vi "禹山溶解氧校准.vi"() -> ()   [LabVIEW 2016, in "斯坦道多参数.lvlib"]
uses:
  <vilib>/Utility/miscctls.llb/LVPointTypeDef.ctl
  <vilib>/Analysis/NI_AALBase.lvlib
  <vilib>/Analysis/NI_AALPro.lvlib
  <vilib>/Utility/config.llb/NI_LVConfig.lvlib
panel:
  out "第二点信号值":dbl
  out "第一点信号值":dbl
  out "通讯状态":string
  in  "盐度自动获取":bool
  in  "大气压补偿":dbl format="%#.2f"
  in  "盐度补偿":dbl format="%#.2f"
  out "DO %":dbl caption="饱和度值" format="%#.2f"
  out "第二点校准值":dbl
  out "第一点校准值":dbl
  out "最小值":sgl format="%.2g"
  out "最大值":sgl format="%.2g"
  in  "校准停止":bool
  in  "校准模式":enum16{"两点校准", "单点校准"}(ring)
  in  "标液2":dbl
  in  "标液1":dbl
  out "波形图表":sgl(graph) caption="历史曲线"
  out "温度测量值":dbl caption="温度" format="%#.2f"
  out "变异系数":dbl format="%.6g"
  out "standard deviation":dbl caption="标准差" format="%0.2f"
  out "mean":dbl caption="均值" format="%0.2f"
  out "提示":string
  in  "校准启动":bool
  out "DO mg/L":dbl caption="测试值" format="%#.2f"
  out "电极斜率":dbl format="%#.6f"
  out "电极零点":dbl format="%#.6f"
  # "溶解氧电极设定"
  # "℃"
  # "%"
  # "mg/L"
  # "kPa"
  # "请选择校准模式:"
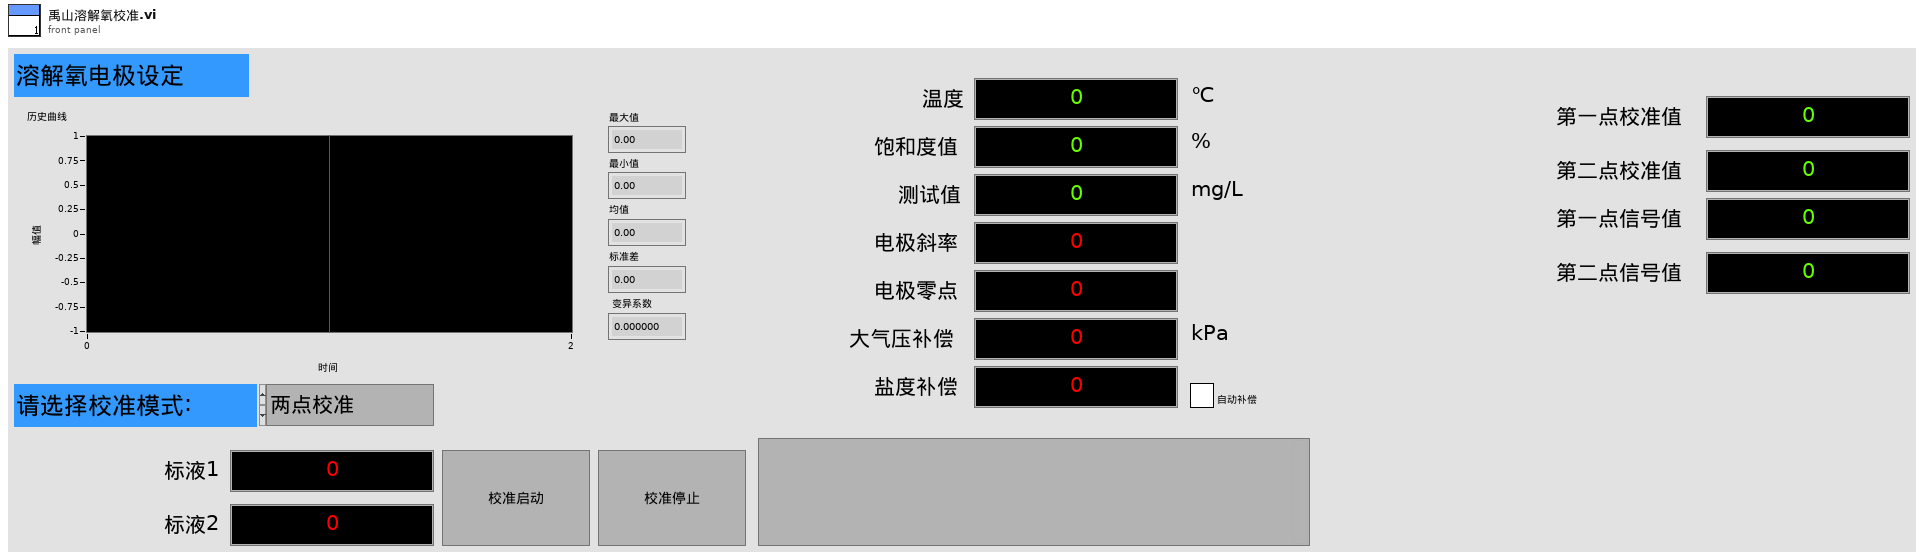
[diagram p1: front panel]
types:
  T1 = typedef "LVPointTypeDef.ctl" = cluster{"Horizontal":i16, "Vertical":i16}
  T2 = typedef "NI_LVConfig.lvlib/Config Data RefNum.ctl" = refnum<k1>
  T3 = enum8{"Enabled", "Disabled", "Disabled and Grayed Out"}
  T4 = cluster{"ph":bool, "DO":bool, "Cond":bool, "Turb":bool, "叶绿素a":bool, "藻密度":bool, "ORP":bool}
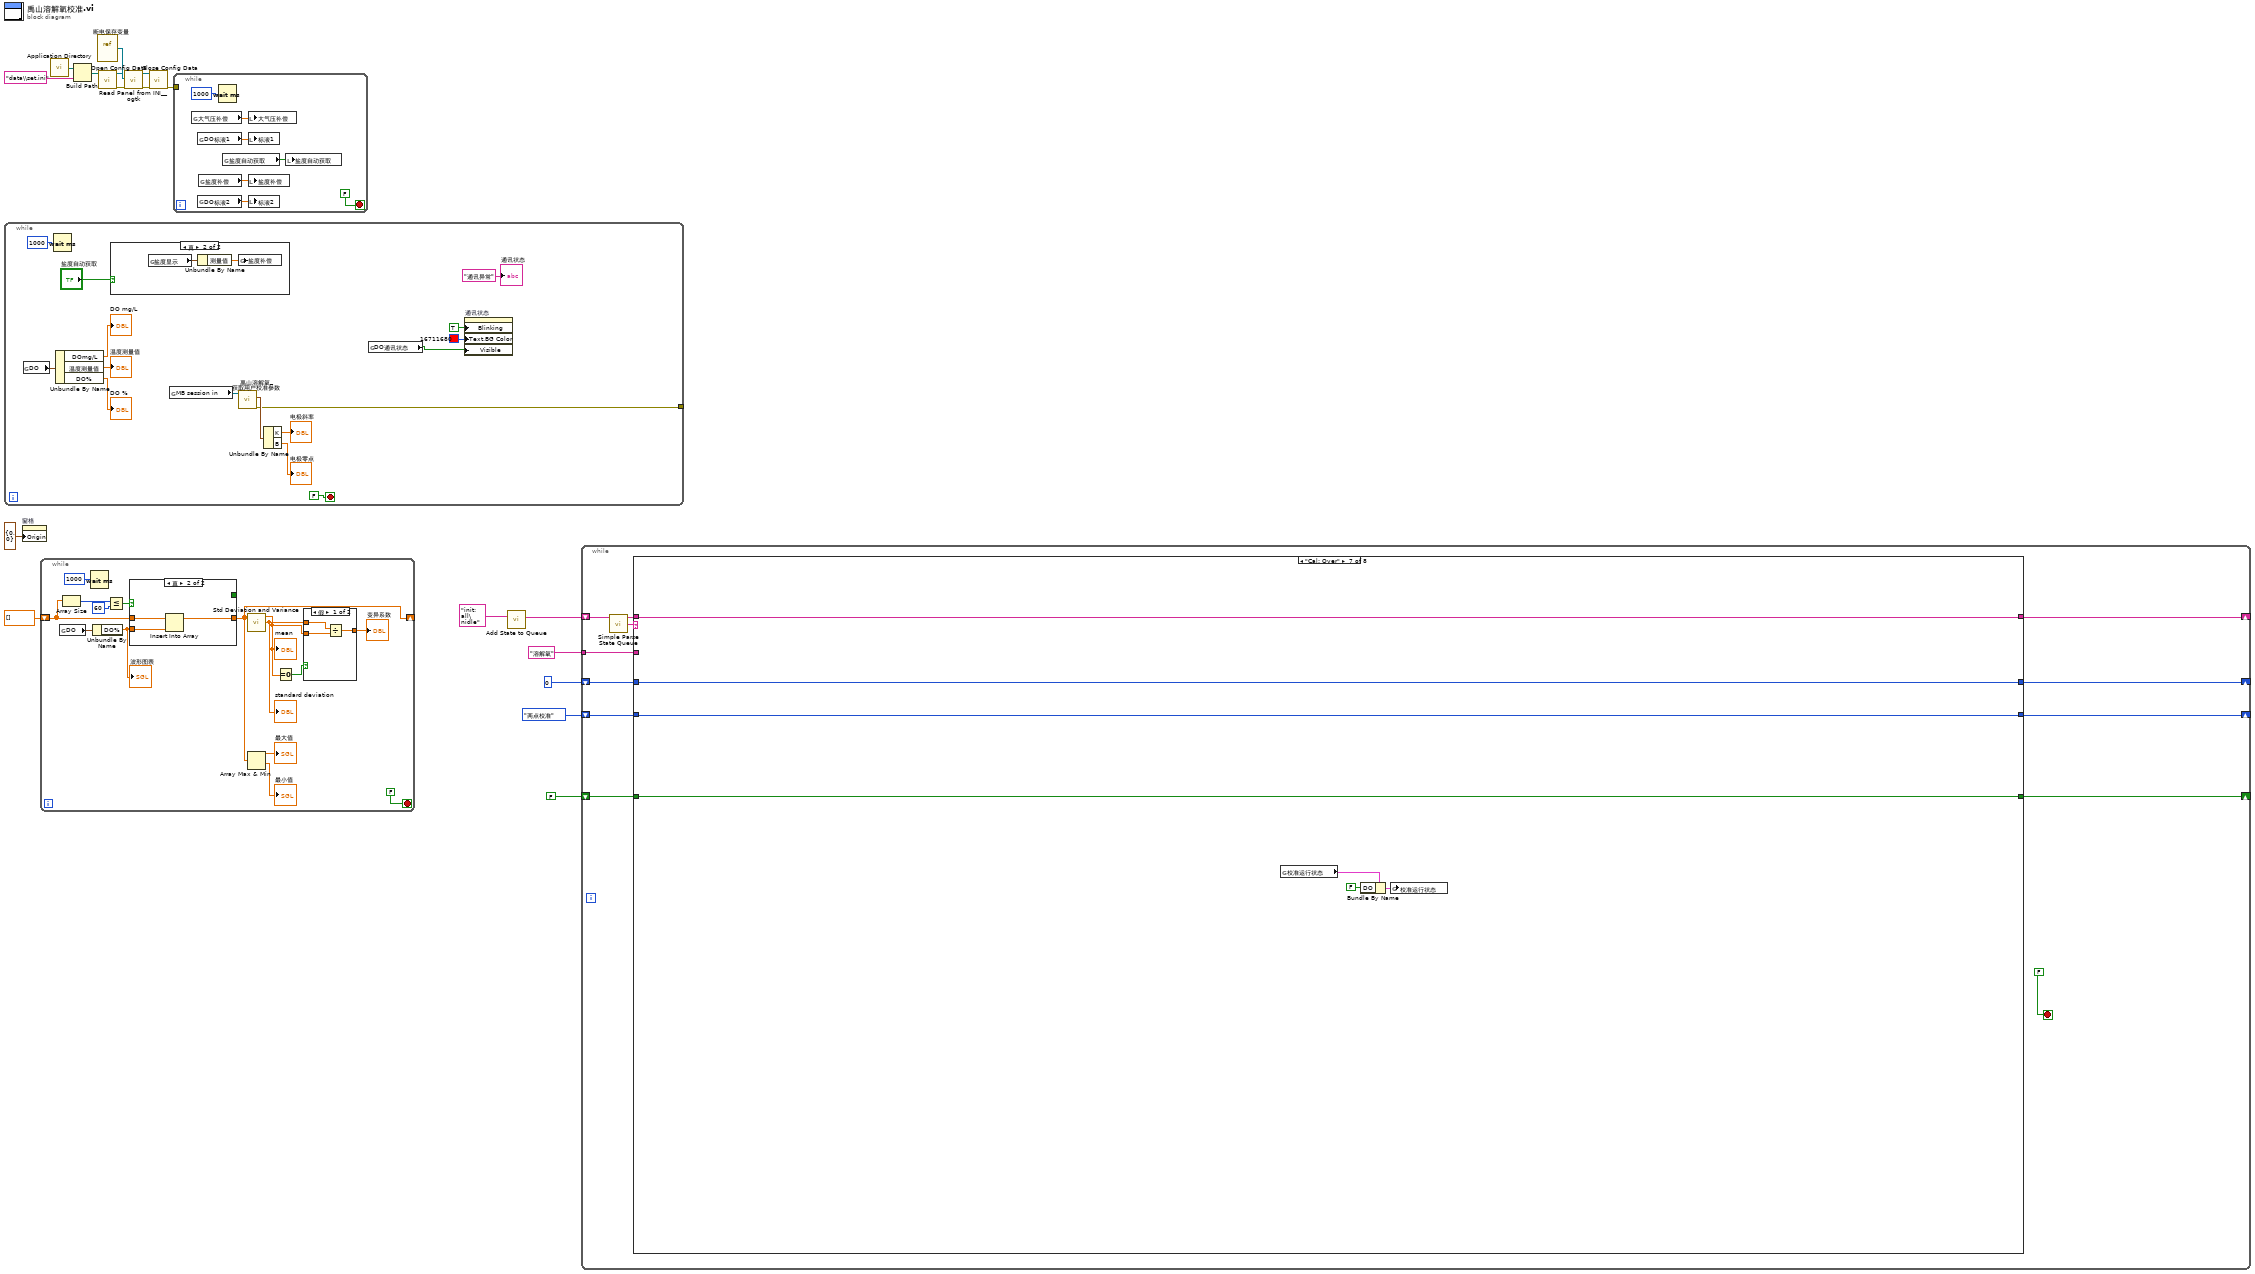
[diagram p0: block diagram]
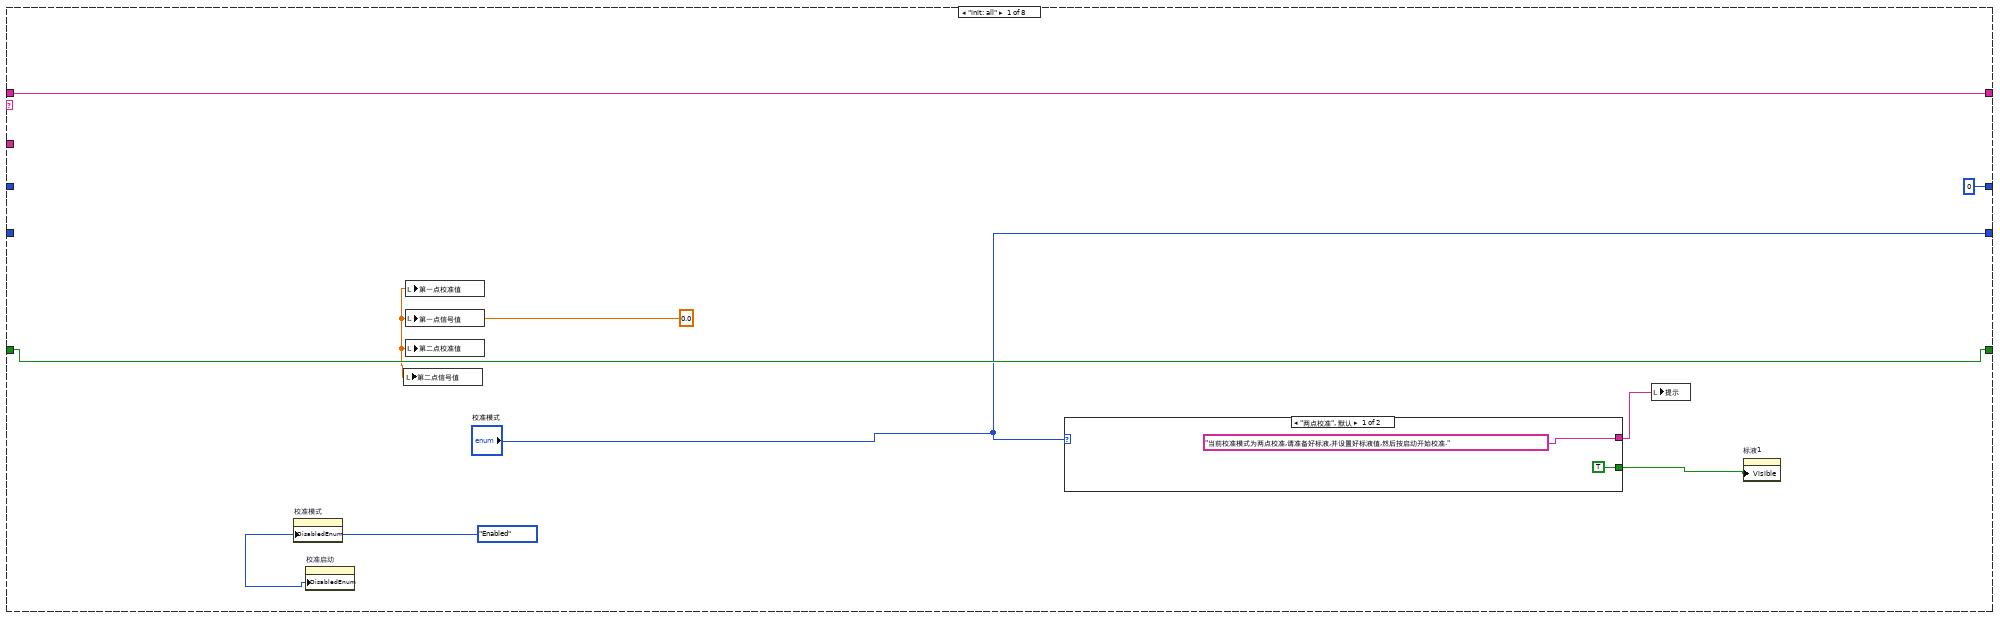
[diagram p2: hidden frame]
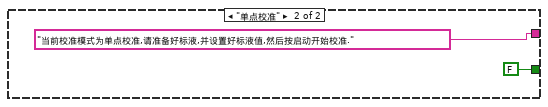
[diagram p3: hidden frame]
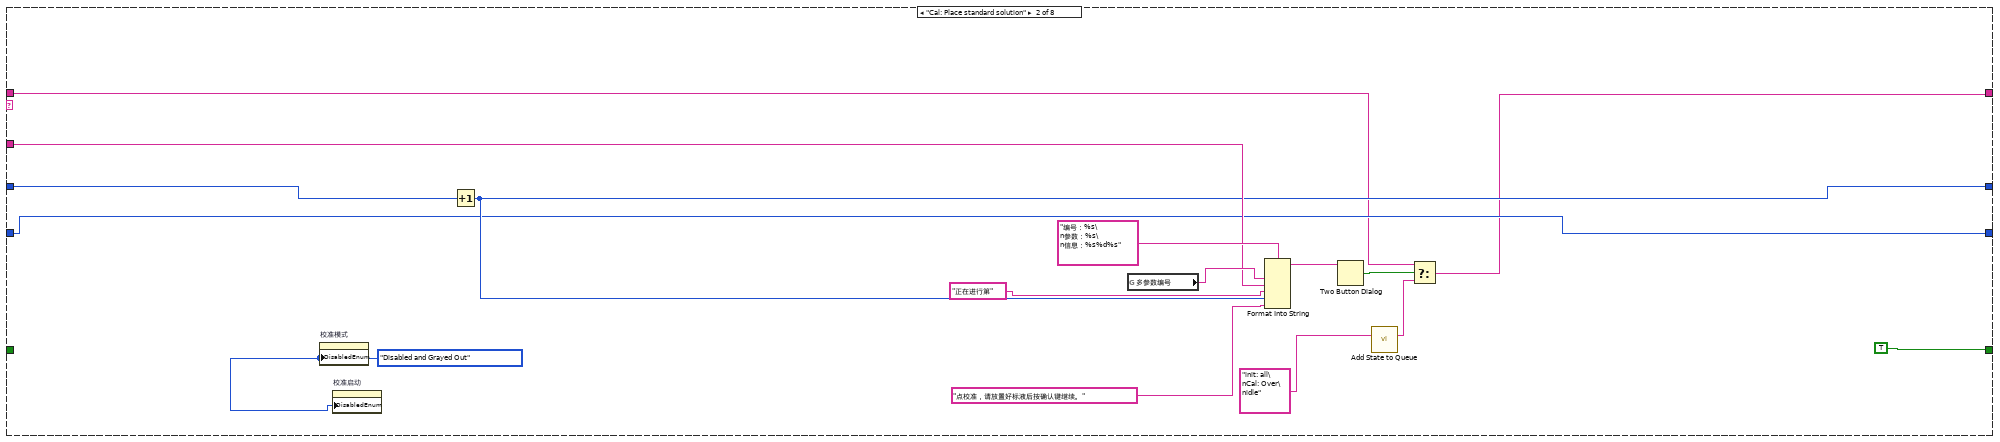
[diagram p4: hidden frame]
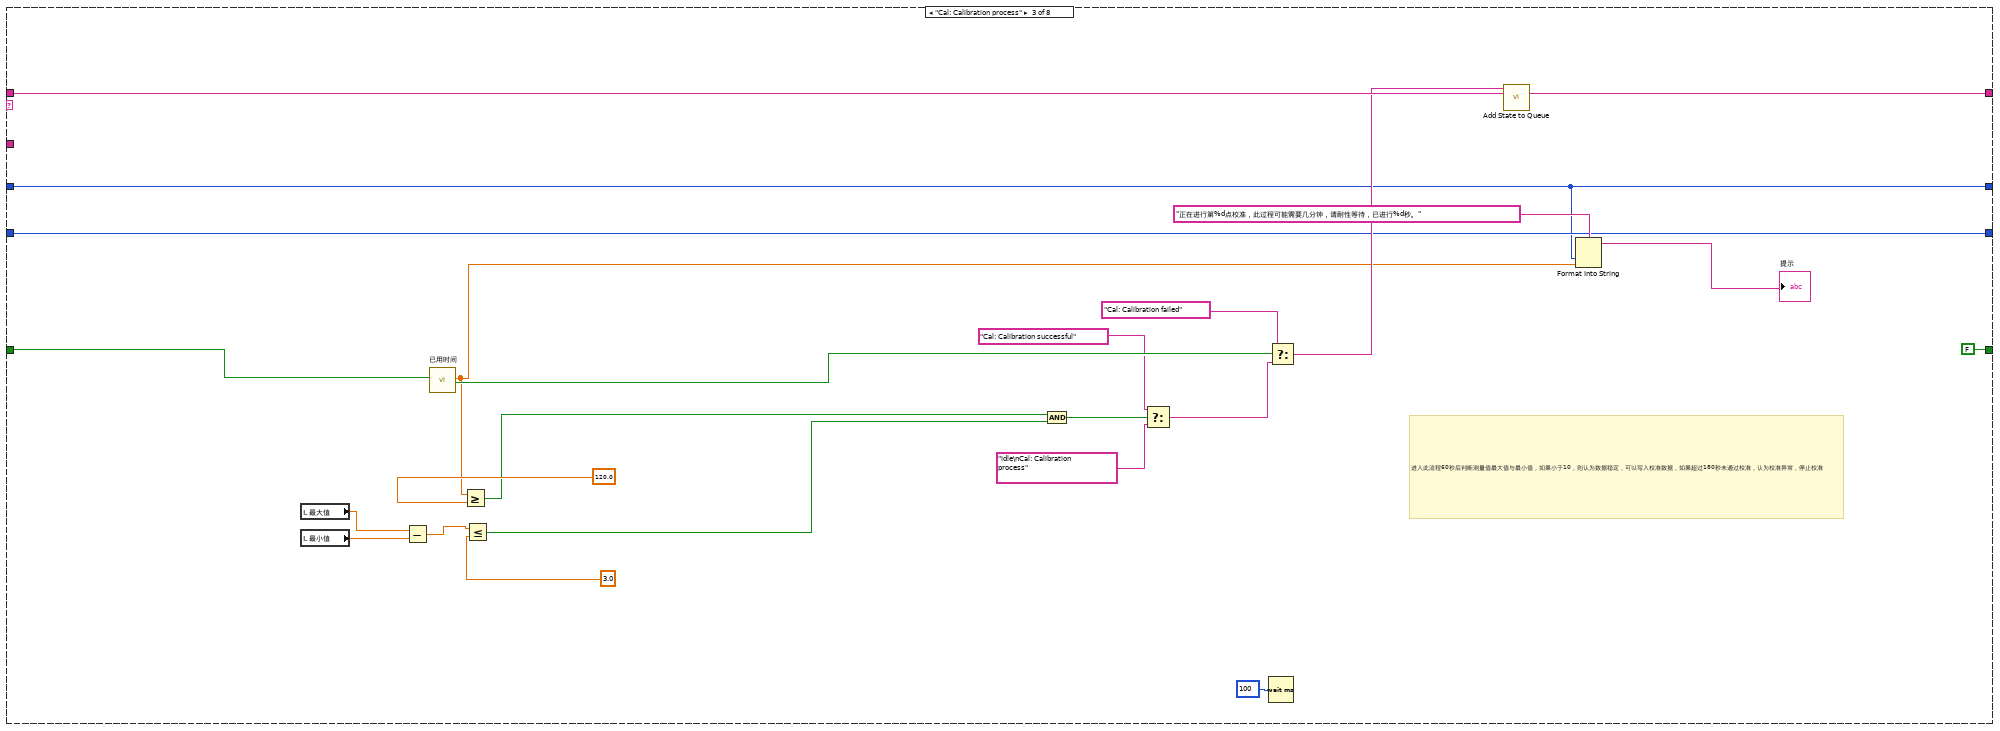
[diagram p5: hidden frame]
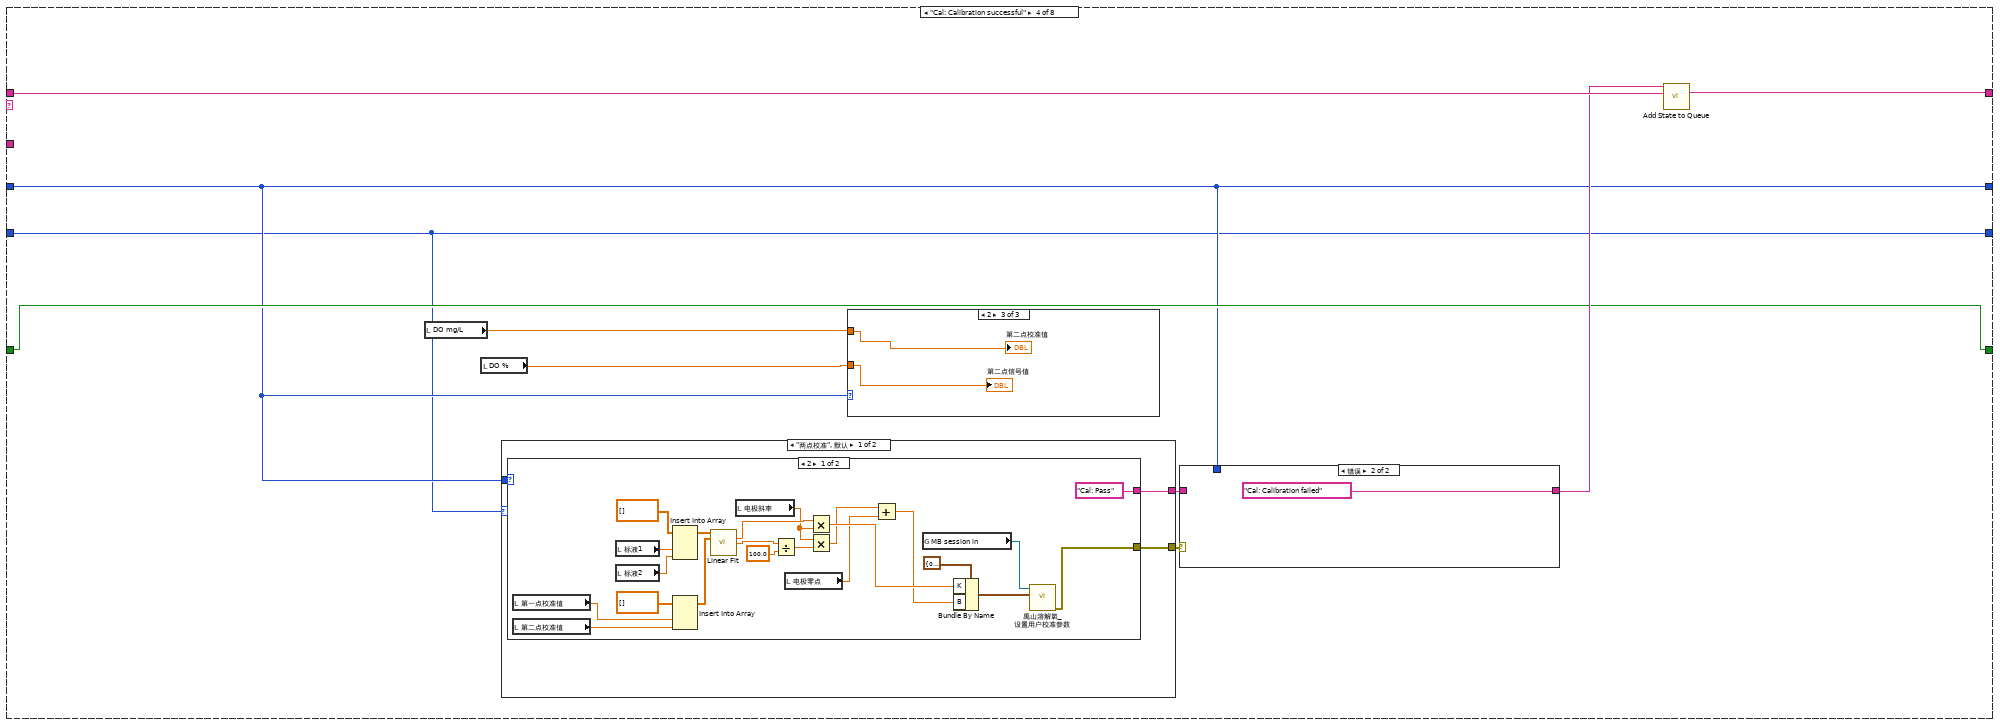
[diagram p6: hidden frame]
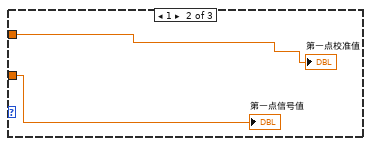
[diagram p8: hidden frame]
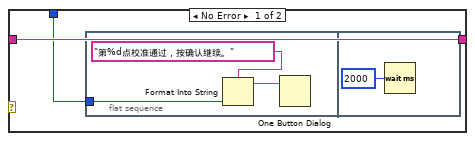
[diagram p9: hidden frame]
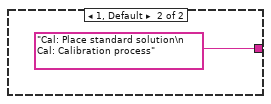
[diagram p10: hidden frame]
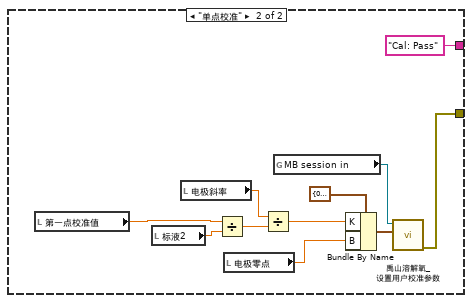
[diagram p11: hidden frame]
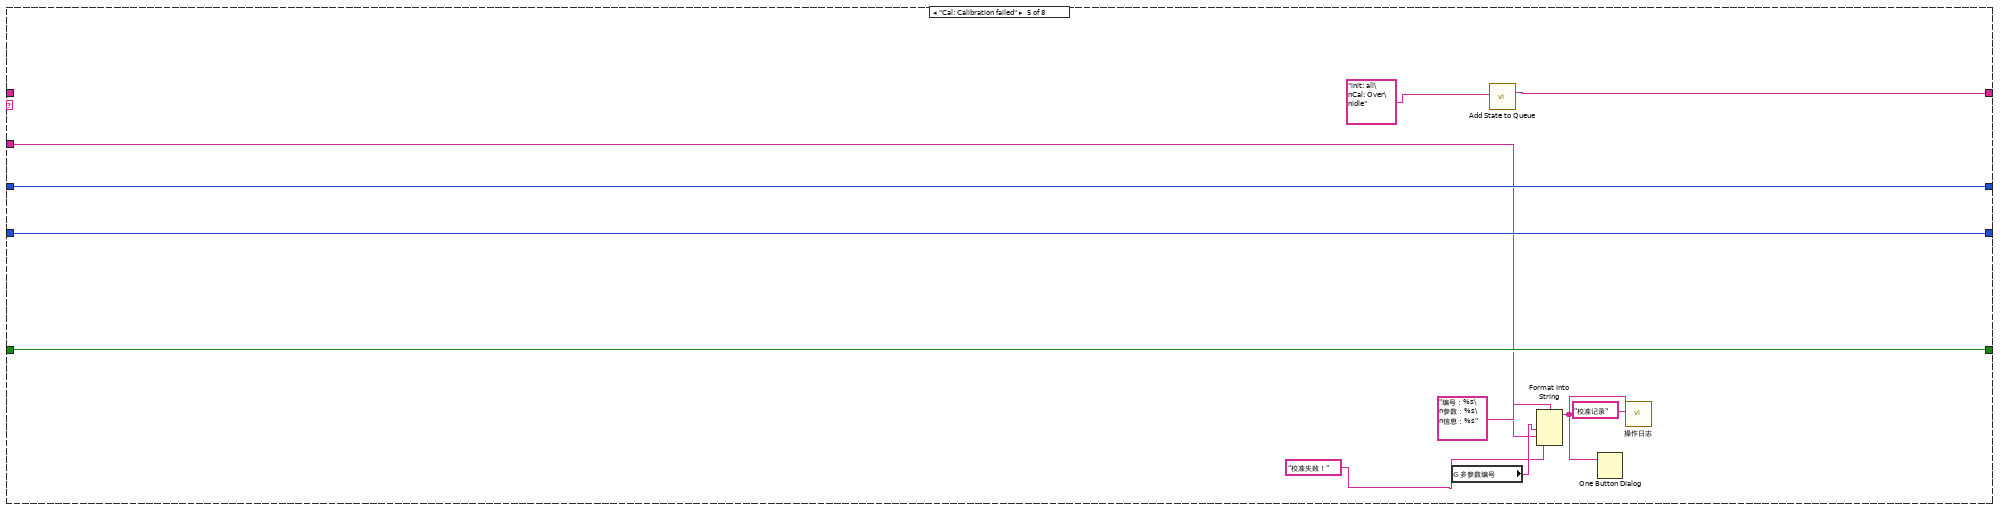
[diagram p12: hidden frame]
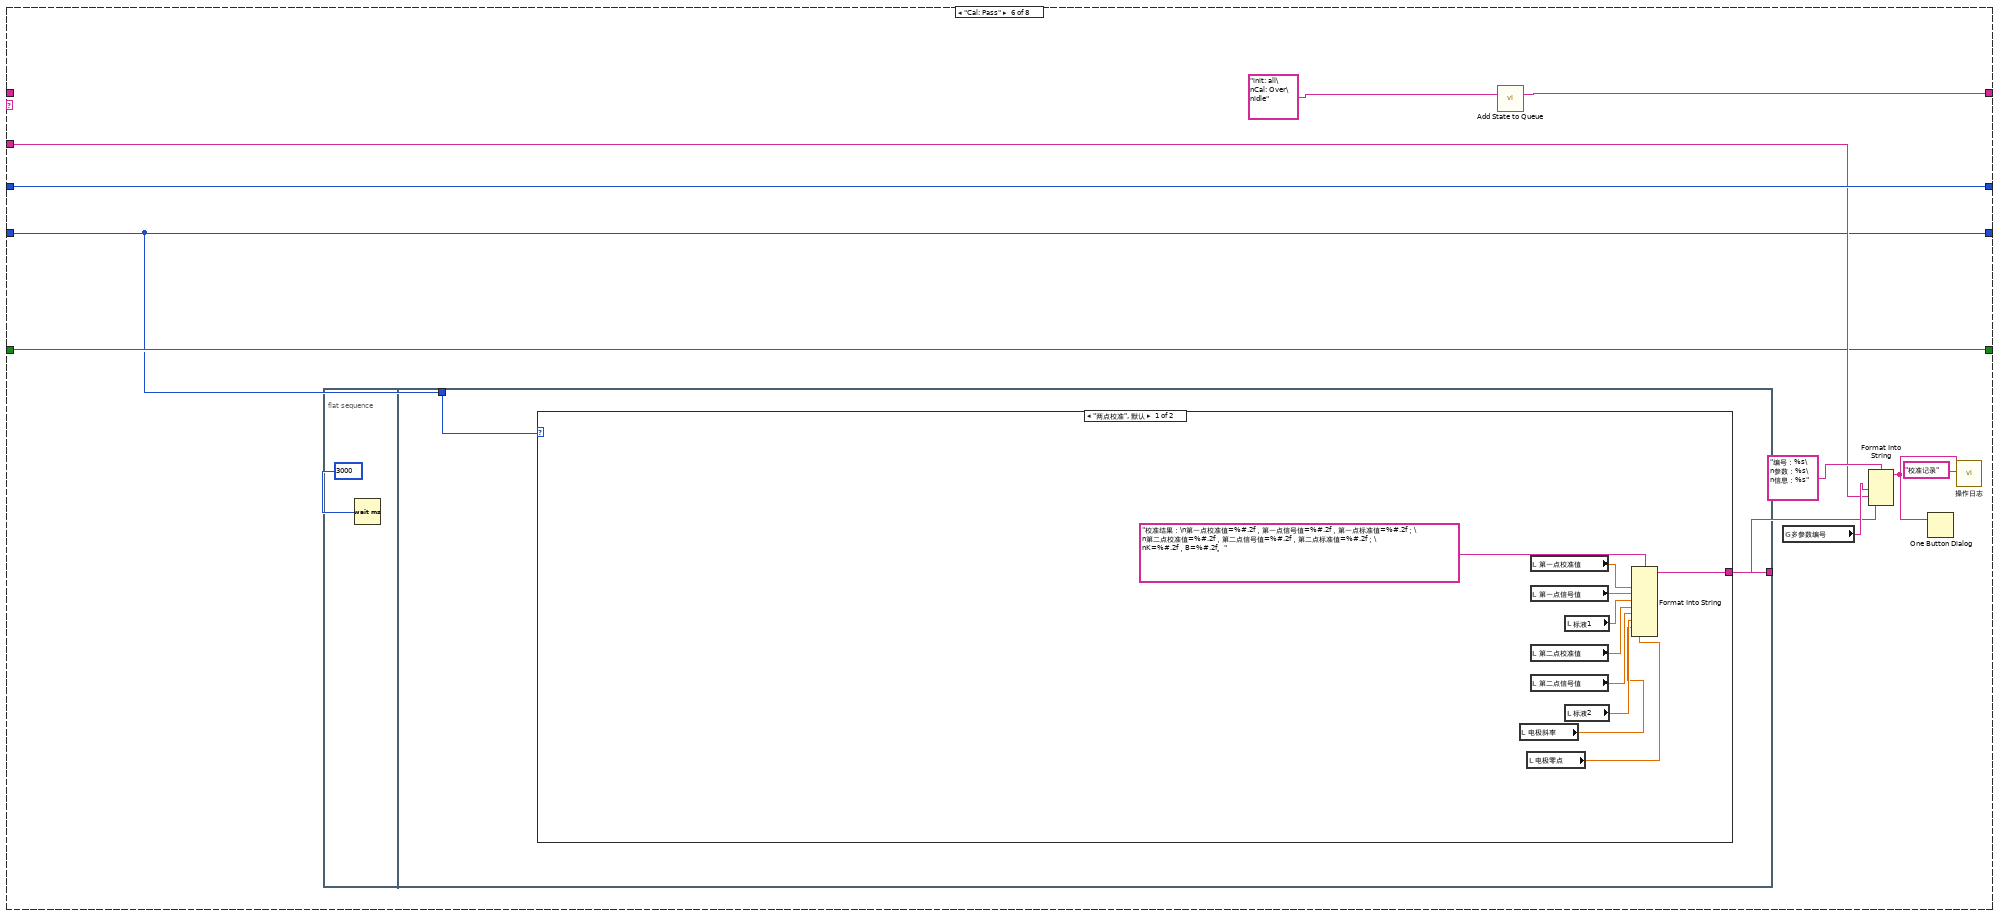
[diagram p13: hidden frame]
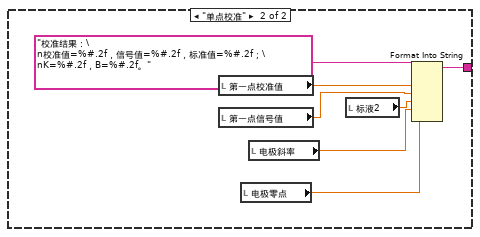
[diagram p14: hidden frame]
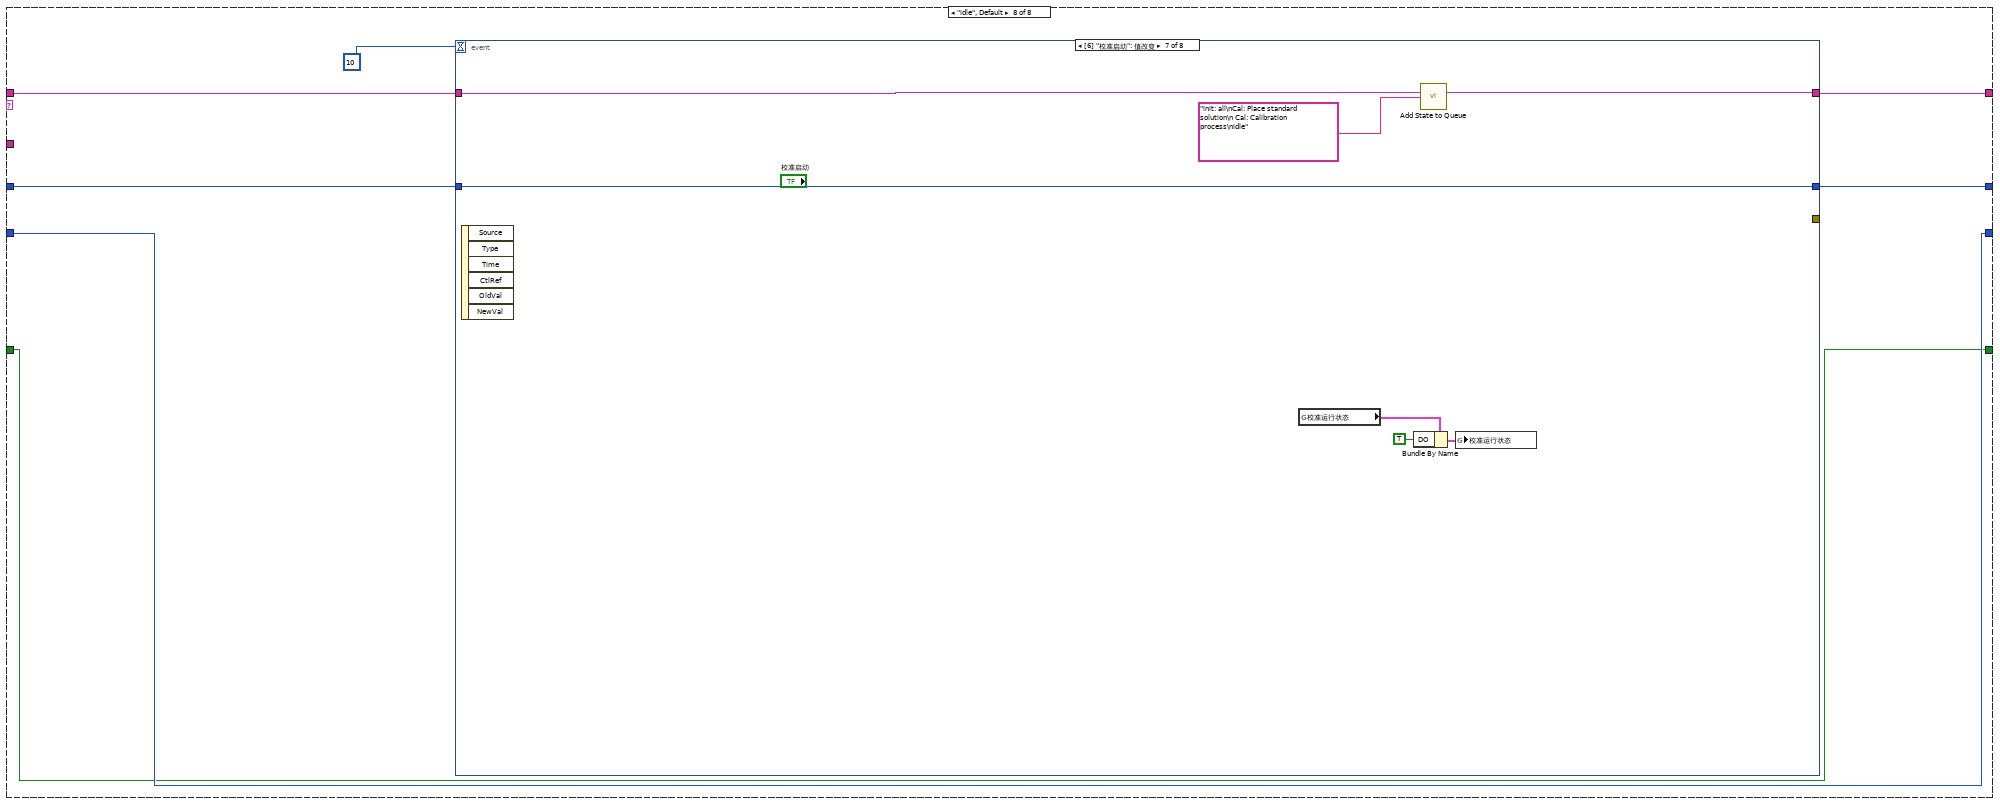
[diagram p15: hidden frame]
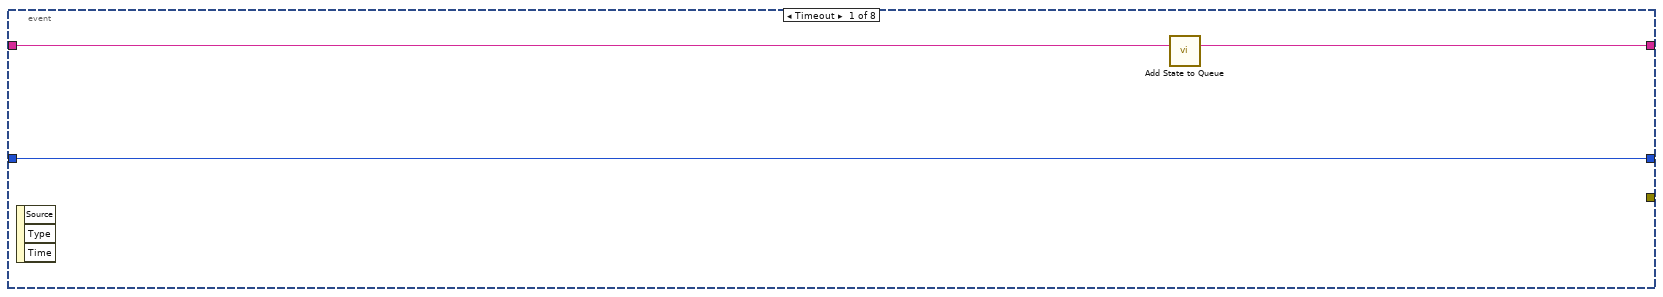
[diagram p16: hidden frame]
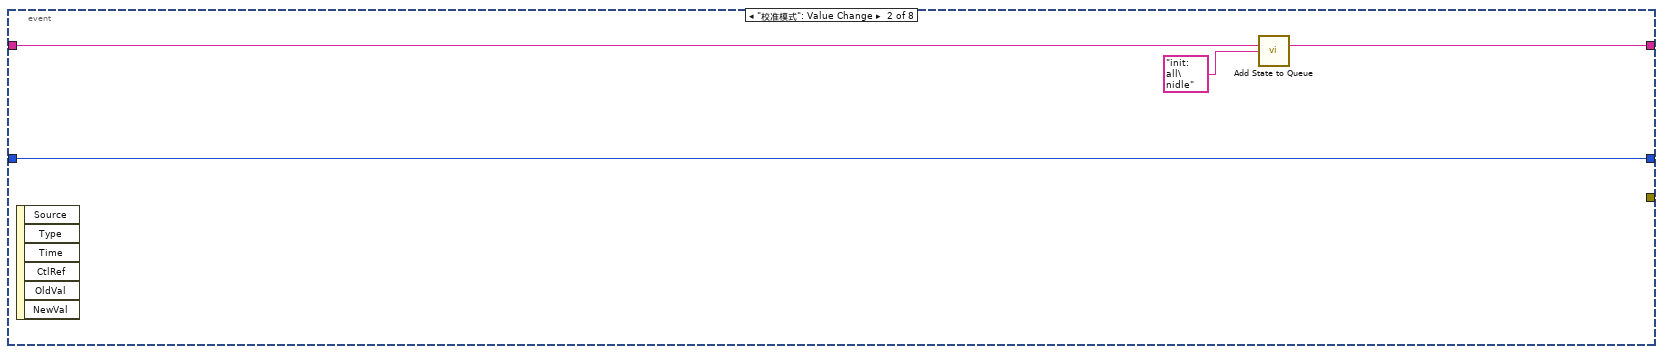
[diagram p17: hidden frame]
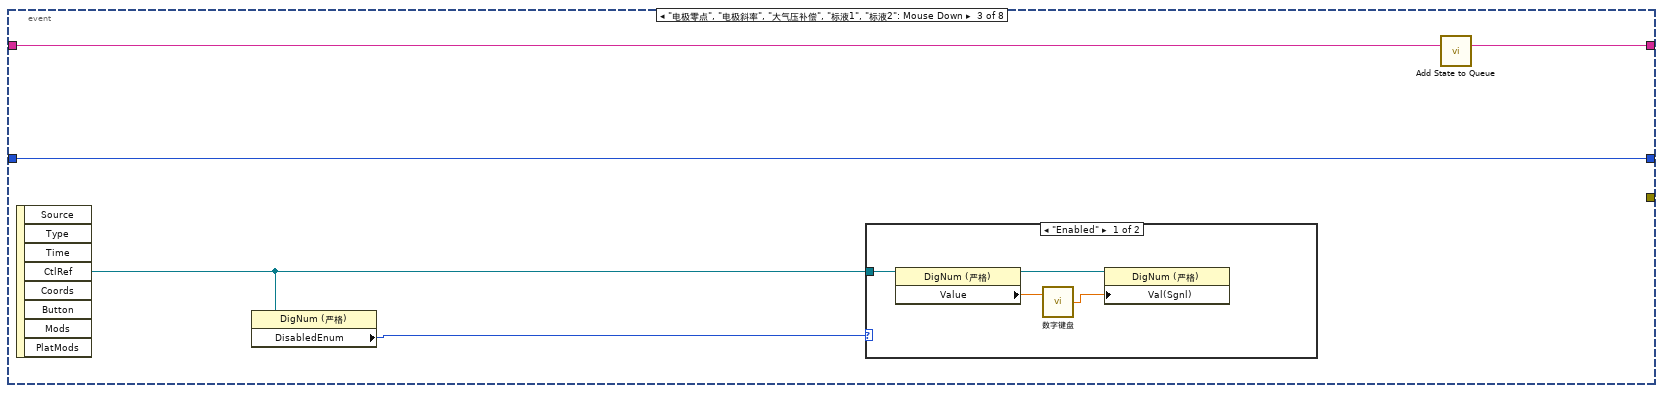
[diagram p18: hidden frame]
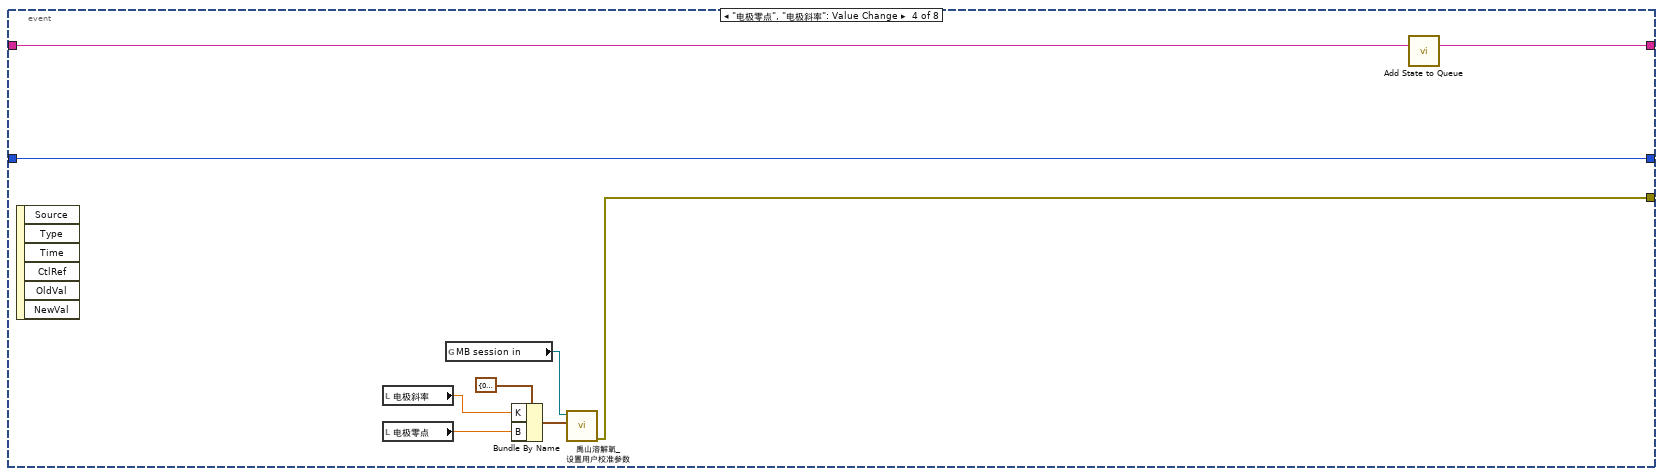
[diagram p20: hidden frame]
diagram:
  n1 = while {
    tunnel: [w28] -> _
    stop <- FALSE stop-if-true
    n2 = global read "禹山过程全局变量.vi" "DO"() -> (w25:cluster{"温度测量值":sgl, "DO%":sgl, "DOmg/L":sgl})
    n3 = Wait (ms)(milliseconds to wait=u32 1000 ("等待时间（毫秒）")) -> ()  [unwired: 1 out]
    n4 = Unbundle By Name(w25) -> ("DOmg/L"=→"DO mg/L":sgl, "温度测量值"=→"温度测量值":sgl, "DO%"=→"DO %":sgl)
    n5 = case shown="真" "盐度自动获取" {
      frame False {
      }
      frame True {
        n6 = global read "多参数全局变量.vi" "盐度显示"() -> (w35:cluster{"温度测量值":sgl, "测量值":sgl, "温度偏移修正值":sgl})
        n7 = Unbundle By Name(w35) -> ("测量值"=w34:sgl)
        n8 = global write "断电保存变量.vi" "盐度补偿"(w34) -> ()
      }
    }
    n9 = global read "多参数全局变量.vi" "MB session in"() -> (w24:refnum<class "MB_Master.lvclass">)
    n10 = call "禹山溶解氧_获取用户校准参数.vi"("MB session in"=w24) -> ("error out"=w28:errorcluster, "输出值"=w31:cluster{"K":sgl, "B":sgl})  [unwired: 8 in, 1 out]
    n11 = Unbundle By Name(w31) -> ("K"=→"电极斜率":sgl, "B"=→"电极零点":sgl)
    n12 = global read "多参数全局变量.vi" "DO通讯状态"() -> (w18:bool)
    n13 = property on="通讯状态" class="Str"("Blinking"=TRUE ("闪烁"), "Text.BG Color"=u32 16711680, "Visible"=w18) -> ()  [unwired: 2 in, 2 out]
    "通讯状态" <- "通讯异常" ("当前串口")
  }
  n14 = property on="窗格" class="Pane"("Origin"=T1 {"Horizontal"=0, "Vertical"=0} ("原点")) -> ()  [unwired: 2 in, 2 out]
  n15 = while {
    shift-right: [w38] -> _
    shift-left: sgl[] [] -> [w46]
    stop <- FALSE stop-if-true
    n16 = global read "禹山过程全局变量.vi" "DO"() -> (w40:cluster{"温度测量值":sgl, "DO%":sgl, "DOmg/L":sgl})
    n17 = Array Size(array=w46) -> (size(s)=w48:i32)
    n18 = Wait (ms)(milliseconds to wait=u32 1000 ("等待时间（毫秒）")) -> ()  [unwired: 1 out]
    n19 = Unbundle By Name(w40) -> ("DO%"=w39:sgl)
    "波形图表" <- w39
    n20 = Less Or Equal?(x=w48, y=60) -> (x <= y?=w47:bool)
    n21 = case shown="真" w47 {
      tunnel: w46 -> [w59 w62]
      tunnel: w39 -> [w57 w61]
      tunnel: [w55 w60] -> w38
      tunnel: [TRUE _] -> _
      frame False {
        n22 = Replace Array Subset(array=w59, new element=w57) -> (w58:sgl[])  [unwired: 1 in]
        n23 = Rotate 1D Array(1:w58, 2:-1 ("n")) -> (0:w55:sgl[])
      }
      frame True {
        n24 = Insert Into Array(array=w62, new element=w61) -> (w60:sgl[])  [unwired: 1 in]
      }
    }
    n25 = call <vilib>:"Std Deviation and Variance.vi"("X"=w38) -> ("mean"=w41:dbl, "standard deviation"=w42:dbl)  [unwired: 1 in, 1 out]
    "standard deviation" <- w42
    "mean" <- w41
    n26 = Array Max & Min(array=w38) -> (max value=→"最大值":sgl, min value=→"最小值":sgl)  [unwired: 2 out]
    n27 = Equal To 0?(x=w41) -> (x = 0?=w45:bool)
    n28 = case shown="假" w45 {
      tunnel: w42 -> [w53 _]
      tunnel: [w52 _] -> w44
      tunnel: w41 -> [w51 _]
      frame False {
        n29 = Divide(x=w53, y=w51) -> (x/y=w52:dbl)
      }
      frame True {
      }
    }
    "变异系数" <- w44
  }
  n30 = call <vilib>:"Application Directory.vi"() -> ("Application Directory"=w12:path)
  n31 = Build Path(base path=w12, name or relative path="data\\set.ini" ("名称或相对路径")) -> (appended path=w13:path)
  n32 = vi-ref "断电保存变量.vi"() -> (w15:refnum<vi>)
  n33 = call <vilib>:"Open Config Data.vi"("configuration file path"=w13) -> ("error out"=w9:errorcluster, "refnum"=w8:T2)  [unwired: 8 in, 1 out]
  n34 = call <userlib>:"Read Panel from INI__ogtk.vi"("error in (no error)"=w9, "VI ref"=w15, "refnum"=w8) -> ("error out"=w11:errorcluster, "refnum out"=w10:T2)  [unwired: 7 in]
  n35 = call <vilib>:"Close Config Data.vi"("error in (no error)"=w11, "refnum"=w10) -> ("error out"=w7:errorcluster)  [unwired: 8 in, 1 out]
  n36 = while {
    tunnel: w7 -> [_]
    stop <- FALSE stop-if-true
    n37 = global read "断电保存变量.vi" "大气压补偿"() -> (w65:dbl)
    n38 = global read "断电保存变量.vi" "DO标液1"() -> (w67:dbl)
    n39 = global read "断电保存变量.vi" "DO标液2"() -> (w66:dbl)
    n40 = global read "断电保存变量.vi" "盐度补偿"() -> (w63:dbl)
    n41 = Wait (ms)(milliseconds to wait=u32 1000 ("等待时间（毫秒）")) -> ()  [unwired: 1 out]
    n42 = global read "断电保存变量.vi" "盐度自动获取"() -> (w64:bool)
    n43 = local write "大气压补偿"(w65) -> ()
    n44 = local write "标液1"(w67) -> ()
    n45 = local write "盐度补偿"(w63) -> ()
    n46 = local write "标液2"(w66) -> ()
    n47 = local write "盐度自动获取"(w64) -> ()
  }
  n48 = call "Add State to Queue.vi"("State(s) In (\"\")"="init: all\nidle" ("State(s) In (\"\")")) -> ("States Out"=w5:string)  [unwired: 14 in]
  n49 = while {
    shift-right: [w77] -> _
    shift-left: w5 -> [w81]
    shift-right: [w74] -> _
    shift-left: 0 -> [w76]
    tunnel: "溶解氧" ("State(s) In (\"\")") -> [w75]
    shift-right: [w72] -> _
    shift-left: enum16{"两点校准", "单点校准"}."两点校准" ("校准模式") -> [w73]
    shift-right: [w70] -> _
    shift-left: FALSE -> [w71]
    stop <- FALSE stop-if-true
    n50 = call "Simple Parse State Queue.vi"("State Queue"=w81) -> ("Remain States"=w78:string, "Next State"=w79:string)  [unwired: 13 in]
    n51 = case shown="\"Cal: Over\"" w79 {
      tunnel: w78 -> [w89 w97 w128 w141 _ _ w240 w247]
      tunnel: [w89 w96 w127 w140 w199 w204 w240 w246] -> w77
      tunnel: w76 -> [_ w105 w112 w135 w202 w213 w239 w244]
      tunnel: w75 -> [_ w106 _ _ w193 w209 _ _]
      tunnel: [0 w103 w112 w135 w202 w213 w239 w245] -> w74
      tunnel: w73 -> [_ w102 w113 w134 w201 w205 w238 w243]
      tunnel: ["校准模式" w102 w113 w134 w201 w205 w238 w243] -> w72
      tunnel: w71 -> [w86 _ w115 w136 w200 w208 w237 w241]
      tunnel: [w86 TRUE FALSE w136 w200 w208 w237 w241] -> w70
      frame "init: all" {
        w84 = T3."Enabled" ("禁用")
        w85 = 0.0 ("第一点校准值")
        n52 = property on="校准模式" class="Enum (严格)"("DisabledEnum"=w84) -> ()  [unwired: 2 in, 2 out]
        n53 = property on="校准启动" class="Bool"("DisabledEnum"=w84) -> ()  [unwired: 2 in, 2 out]
        n54 = local write "第二点信号值"(w85) -> ()
        n55 = local write "第一点校准值"(w85) -> ()
        n56 = local write "第一点信号值"(w85) -> ()
        n57 = local write "第二点校准值"(w85) -> ()
        n58 = case shown="\"两点校准\", 默认" "校准模式" {
          tunnel: ["当前校准模式为两点校准,请准备好标液,并设置好标液值,然后按启动开始校准." ("提示") "当前校准模式为单点校准,请准备好标液,并设置好标液值,然后按启动开始校准." ("提示")] -> w88
          tunnel: [TRUE ("可见") FALSE ("可见")] -> w82
          frame "两点校准", Default {
          }
          frame "单点校准" {
          }
        }
        n59 = local write "提示"(w88) -> ()
        n60 = property on="标液1" class="DigNum (严格)"("Visible"=w82) -> ()  [unwired: 2 in, 2 out]
      }
      frame "Cal: Place standard solution" {
        w95 = T3."Disabled and Grayed Out" ("禁用")
        n61 = property on="校准模式" class="Enum (严格)"("DisabledEnum"=w95) -> ()  [unwired: 2 in, 2 out]
        n62 = property on="校准启动" class="Bool"("DisabledEnum"=w95) -> ()  [unwired: 2 in, 2 out]
        n63 = Increment(x=w105) -> (x+1=w103:i32)
        n64 = global read "多参数全局变量.vi" "多参数编号"() -> (w108:string)
        n65 = Format Into String(format string="编号：%s\n参数：%s\n信息：%s%d%s" ("格式字符串"), w108, w106, "正在进行第" ("消息"), w103, "点校准，请放置好标液后按确认键继续。" ("消息")) -> (resulting string=w100:string)  [unwired: 2 in, 1 out]
        n66 = Two Button Dialog(message=w100) -> (T button?=w99:bool)  [unwired: 2 in]
        n67 = call "Add State to Queue.vi"("State(s) In (\"\")"="init: all\nCal: Over\nidle" ("State(s) In (\"\")")) -> ("States Out"=w98:string)  [unwired: 14 in]
        n68 = Select(t=w97, s=w99, f=w98) -> (s? t:f=w96:string)
      }
      frame "Cal: Calibration process" {
        # "进入此流程60秒后判断测量值最大值与最小值，如果小于10，则认为数据稳定，可以写入校准数据，如果超过180秒未通过校准，认为校准异常，停止校准"
        n69 = local read "最大值"() -> (w132:sgl)
        n70 = local read "最小值"() -> (w131:sgl)
        n71 = Subtract(x=w132, y=w131) -> (x-y=w133:sgl)
        n72 = call "已用时间"("Reset"=w115) -> ("Elapsed Time (s)"=w111:dbl, "Time has Elapsed"=w129:bool)  [unwired: 11 in, 6 out]
        n73 = Greater Or Equal?(x=w111, y=120.0) -> (x >= y?=w124:bool)
        n74 = Less Or Equal?(x=w133, y=3.0) -> (x <= y?=w120:bool)
        n75 = And(x=w124, y=w120) -> (x .and. y?=w121:bool)
        n76 = Select(t="Cal: Calibration successful" ("State(s) In (\"\")"), s=w121, f="idle\nCal: Calibration process" ("State(s) In (\"\")")) -> (s? t:f=w119:string)
        n77 = Wait (ms)(milliseconds to wait=u32 100 ("等待时间（毫秒）")) -> ()  [unwired: 1 out]
        n78 = Select(t="Cal: Calibration failed" ("State(s) In (\"\")"), s=w129, f=w119) -> (s? t:f=w118:string)
        n79 = call "Add State to Queue.vi"("State(s) In Front (\"\")"=w118, "State(s) In (\"\")"=w128) -> ("States Out"=w127:string)  [unwired: 13 in]
        n80 = Format Into String(format string="正在进行第%d点校准，此过程可能需要几分钟，请耐性等待，已进行%d秒。" ("格式字符串"), w112, w111) -> (resulting string=→"提示":string)  [unwired: 2 in, 1 out]
      }
      frame "Cal: Calibration successful" {
        n81 = local read "DO mg/L"() -> (w137:dbl)
        n82 = local read "DO %"() -> (w138:dbl)
        n83 = case shown="\"两点校准\", 默认" w134 {
          tunnel: [w157 w181] -> w143
          tunnel: [w156 "Cal: Pass" ("State(s) In (\"\")")] -> w142
          tunnel: w135 -> [w155 _]
          frame "两点校准", Default {
            n84 = case shown="2" w155 {
              tunnel: [w158 _] -> w157
              tunnel: ["Cal: Pass" ("State(s) In (\"\")") "Cal: Place standard solution\n Cal: Calibration process" ("State(s) In (\"\")")] -> w156
              frame 2 {
                n85 = local read "第一点校准值"() -> (w177:dbl)
                n86 = local read "第二点校准值"() -> (w176:dbl)
                n87 = local read "标液1"() -> (w174:dbl)
                n88 = local read "标液2"() -> (w173:dbl)
                n89 = Insert Into Array(array=dbl[] [] ("Weight"), new element #1=w174, new element #2=w173) -> (w172:dbl[])  [unwired: 1 in]
                n90 = Insert Into Array(array=dbl[] [] ("Weight"), new element #1=w177, new element #2=w176) -> (w171:dbl[])  [unwired: 1 in]
                n91 = call <vilib>:"Linear Fit.vi"("Y"=w172, "X"=w171) -> ("slope"=w167:dbl, "intercept"=w164:dbl)  [unwired: 9 in, 3 out]
                n92 = local read "电极斜率"() -> (w165:dbl)
                n93 = Divide(x=w164, y=100.0) -> (x/y=w160:dbl)
                n94 = local read "电极零点"() -> (w162:dbl)
                n95 = Multiply(x=w167, y=w165) -> (x*y=w166:dbl)
                n96 = Multiply(x=w165, y=w160) -> (x*y=w163:dbl)
                n97 = Add(x=w163, y=w162) -> (x+y=w161:dbl)
                n98 = global read "多参数全局变量.vi" "MB session in"() -> (w170:refnum<class "MB_Master.lvclass">)
                n99 = Bundle By Name(cluster=cluster{"K":sgl, "B":sgl} {"K"=0.0, "B"=0.0} ("用户校准参数"), "K"=w166, "B"=w161) -> (w169:cluster{"K":sgl, "B":sgl})
                n100 = call "禹山溶解氧_设置用户校准参数.vi"("用户校准参数"=w169, "MB session in"=w170) -> ("error out"=w158:errorcluster)  [unwired: 8 in, 1 out]
              }
              frame 1, Default {
              }
            }
          }
          frame "单点校准" {
            n101 = local read "第一点校准值"() -> (w186:dbl)
            n102 = local read "标液2"() -> (w185:dbl)
            n103 = local read "电极斜率"() -> (w183:dbl)
            n104 = Divide(x=w186, y=w185) -> (x/y=w182:dbl)
            n105 = local read "电极零点"() -> (w187:dbl)
            n106 = Divide(x=w183, y=w182) -> (x/y=w184:dbl)
            n107 = global read "多参数全局变量.vi" "MB session in"() -> (w190:refnum<class "MB_Master.lvclass">)
            n108 = Bundle By Name(cluster=cluster{"K":sgl, "B":sgl} {"K"=0.0, "B"=0.0} ("用户校准参数"), "K"=w184, "B"=w187) -> (w189:cluster{"K":sgl, "B":sgl})
            n109 = call "禹山溶解氧_设置用户校准参数.vi"("用户校准参数"=w189, "MB session in"=w190) -> ("error out"=w181:errorcluster)  [unwired: 8 in, 1 out]
          }
        }
        n110 = case shown="2" w135 {
          tunnel: w138 -> [_ w145 w147]
          tunnel: w137 -> [_ w144 w146]
          frame 0, Default {
          }
          frame 1 {
            "第一点信号值" <- w145
            "第一点校准值" <- w144
          }
          frame 2 {
            "第二点信号值" <- w147
            "第二点校准值" <- w146
          }
        }
        n111 = case shown="错误" w143 {
          tunnel: w142 -> [w149 _]
          tunnel: [w149 "Cal: Calibration failed" ("State(s) In (\"\")")] -> w139
          tunnel: w135 -> [w148 _]
          frame No Error {
            n112 = flat-sequence {
              tunnel: w148 -> [w150]
              frame #0 {
                n113 = Format Into String(format string="第%d点校准通过，按确认继续。" ("格式字符串"), w150) -> (resulting string=w152:string)  [unwired: 2 in, 1 out]
                n114 = One Button Dialog(message=w152) -> ()  [unwired: 1 in, 1 out]
              }
              frame #1 {
                n115 = Wait (ms)(milliseconds to wait=u32 2000 ("等待时间（毫秒）")) -> ()  [unwired: 1 out]
              }
            }
          }
          frame Error {
          }
        }
        n116 = call "Add State to Queue.vi"("State(s) In Front (\"\")"=w139, "State(s) In (\"\")"=w141) -> ("States Out"=w140:string)  [unwired: 13 in]
      }
      frame "Cal: Calibration failed" {
        n117 = global read "多参数全局变量.vi" "多参数编号"() -> (w196:string)
        n118 = call "Add State to Queue.vi"("State(s) In (\"\")"="init: all\nCal: Over\nidle" ("State(s) In (\"\")")) -> ("States Out"=w199:string)  [unwired: 14 in]
        n119 = Format Into String(format string="编号：%s\n参数：%s\n信息：%s" ("格式字符串"), w196, w193, "校准失败！" ("消息")) -> (resulting string=w195:string)  [unwired: 2 in, 1 out]
        n120 = One Button Dialog(message=w195) -> ()  [unwired: 1 in, 1 out]
        n121 = call "操作日志.vi"("table"="校准记录", "日志信息"=w195) -> ()  [unwired: 9 in, 1 out]
      }
      frame "Cal: Pass" {
        n122 = flat-sequence {
          tunnel: [w216] -> w206
          tunnel: w205 -> [w215]
          frame #0 {
            n123 = Wait (ms)(milliseconds to wait=u32 3000 ("等待时间（毫秒）")) -> ()  [unwired: 1 out]
          }
          frame #1 {
            n124 = case shown="\"两点校准\", 默认" w215 {
              tunnel: [w226 w233] -> w216
              frame "两点校准", Default {
                n125 = local read "电极斜率"() -> (w218:dbl)
                n126 = local read "电极零点"() -> (w217:dbl)
                n127 = local read "第一点校准值"() -> (w224:dbl)
                n128 = local read "第一点信号值"() -> (w225:dbl)
                n129 = local read "第二点校准值"() -> (w221:dbl)
                n130 = local read "第二点信号值"() -> (w220:dbl)
                n131 = local read "标液1"() -> (w222:dbl)
                n132 = local read "标液2"() -> (w219:dbl)
                n133 = Format Into String(format string="校准结果：\n第一点校准值=%#.2f，第一点信号值=%#.2f，第一点标准值=%#.2f；\n第二点校准值=%#.2f，第二点信号值=%#.2f，第二点标准值=%#.2f；\nK=%#.2f，B=%#.2f。" ("提示"), w224, w225, w222, w221, w220, w219, w218, w217) -> (resulting string=w226:string)  [unwired: 2 in, 1 out]
              }
              frame "单点校准" {
                n134 = local read "第一点校准值"() -> (w232:dbl)
                n135 = local read "第一点信号值"() -> (w230:dbl)
                n136 = local read "电极零点"() -> (w227:dbl)
                n137 = local read "电极斜率"() -> (w228:dbl)
                n138 = local read "标液2"() -> (w229:dbl)
                n139 = Format Into String(format string="校准结果：\n校准值=%#.2f，信号值=%#.2f，标准值=%#.2f；\nK=%#.2f，B=%#.2f。" ("提示"), w232, w230, w229, w228, w227) -> (resulting string=w233:string)  [unwired: 2 in, 1 out]
              }
            }
          }
        }
        n140 = call "Add State to Queue.vi"("State(s) In (\"\")"="init: all\nCal: Over\nidle" ("State(s) In (\"\")")) -> ("States Out"=w204:string)  [unwired: 14 in]
        n141 = global read "多参数全局变量.vi" "多参数编号"() -> (w210:string)
        n142 = Format Into String(format string="编号：%s\n参数：%s\n信息：%s" ("格式字符串"), w210, w209, w206) -> (resulting string=w207:string)  [unwired: 2 in, 1 out]
        n143 = One Button Dialog(message=w207) -> ()  [unwired: 1 in, 1 out]
        n144 = call "操作日志.vi"("table"="校准记录", "日志信息"=w207) -> ()  [unwired: 9 in, 1 out]
      }
      frame "Cal: Over" {
        n145 = global read "多参数全局变量.vi" "校准运行状态"() -> (w235:T4)
        n146 = Bundle By Name(cluster=w235, "DO"=FALSE) -> (w236:T4)
        n147 = global write "多参数全局变量.vi" "校准运行状态"(w236) -> ()
      }
      frame "idle", Default {
        n148 = event shown="[6] \"校准启动\": 值改变" {
          selector: _ -> [_ _ _ _ _ _ _ _]
          dyn-events: _ -> [_ _ _ _ _ _ _ _]
          timeout: 10 -> [_ _ _ _ _ _ _ _]
          tunnel: [_ _ _ w265 _ _ _ _] -> _
          tunnel: w247 -> [w250 w254 w257 w264 w273 w295 w310 _]
          tunnel: [w249 w253 w258 w271 w274 w297 w309 w312] -> w246
          tunnel: [w248 w251 w259 w272 w275 w296 w307 w313] -> w245
          tunnel: w244 -> [w248 w251 w259 w272 w275 w296 w307 w313]
          event Timeout {
            n149 = event-data() -> ()  [unwired: 1 in, 3 out]
            n150 = call "Add State to Queue.vi"("State(s) In (\"\")"=w250) -> ("States Out"=w249:string)  [unwired: 14 in]
          }
          event "校准模式": Value Change {
            n151 = event-data() -> ()  [unwired: 1 in, 6 out]
            n152 = call "Add State to Queue.vi"("State(s) In (\"\")"=w254, "State(s) At Back (\"\")"="init: all\nidle" ("State(s) In (\"\")")) -> ("States Out"=w253:string)  [unwired: 13 in]
          }
          event "电极零点", "电极斜率", "大气压补偿", "标液1", "标液2": Mouse Down {
            n153 = event-data() -> ("CtlRef"=w256:refnum<vi>)  [unwired: 1 in, 7 out]
            n154 = property class="DigNum (严格)"(reference=w256) -> ("DisabledEnum"=w255:T3)  [unwired: 1 in, 2 out]
            n155 = case shown="\"Enabled\"" w255 {
              tunnel: w256 -> [w263 _]
              frame "Enabled" {
                n156 = property class="DigNum (严格)"(reference=w263) -> (reference out=w260:refnum<vi>, "Value"=w261:dbl)  [unwired: 1 in, 1 out]
                n157 = call "数字键盘.vi"("OldNumber"=w261) -> ("NewNumber"=w262:dbl)  [unwired: 1 in]
                n158 = property class="DigNum (严格)"(reference=w260, "Val(Sgnl)"=w262) -> ()  [unwired: 1 in, 2 out]
              }
              frame "Disabled", Default {
              }
            }
            n159 = call "Add State to Queue.vi"("State(s) In (\"\")"=w257) -> ("States Out"=w258:string)  [unwired: 14 in]
          }
          event "电极零点", "电极斜率": Value Change {
            n160 = event-data() -> ()  [unwired: 1 in, 6 out]
            n161 = local read "电极斜率"() -> (w268:dbl)
            n162 = local read "电极零点"() -> (w267:dbl)
            n163 = global read "多参数全局变量.vi" "MB session in"() -> (w266:refnum<class "MB_Master.lvclass">)
            n164 = Bundle By Name(cluster=cluster{"K":sgl, "B":sgl} {"K"=0.0, "B"=0.0} ("用户校准参数"), "K"=w268, "B"=w267) -> (w269:cluster{"K":sgl, "B":sgl})
            n165 = call "禹山溶解氧_设置用户校准参数.vi"("用户校准参数"=w269, "MB session in"=w266) -> ("error out"=w265:errorcluster)  [unwired: 8 in, 1 out]
            n166 = call "Add State to Queue.vi"("State(s) In (\"\")"=w264) -> ("States Out"=w271:string)  [unwired: 14 in]
          }
          event "标液1", "标液2", "大气压补偿", "盐度补偿", "盐度自动获取": Value Change {
            n167 = event-data() -> ()  [unwired: 1 in, 6 out]
            n168 = flat-sequence {
              frame #0 {
                n169 = local read "盐度自动获取"() -> (w276:bool)
                n170 = global write "断电保存变量.vi" "盐度补偿"("盐度补偿") -> ()
                n171 = global write "断电保存变量.vi" "DO标液1"("标液1") -> ()
                n172 = global write "断电保存变量.vi" "DO标液2"("标液2") -> ()
                n173 = global write "断电保存变量.vi" "大气压补偿"("大气压补偿") -> ()
                n174 = global write "断电保存变量.vi" "盐度自动获取"(w276) -> ()
              }
              frame #1 {
                n175 = call <vilib>:"Application Directory.vi"() -> ("Application Directory"=w290:path)
                n176 = Build Path(base path=w290, name or relative path="data\\set.ini" ("名称或相对路径")) -> (appended path=w289:path)
                n177 = call <vilib>:"Open Config Data.vi"("configuration file path"=w289) -> ("error out"=w293:errorcluster, "refnum"=w294:T2)  [unwired: 8 in, 1 out]
                n178 = vi-ref "断电保存变量.vi"() -> (w287:refnum<vi>)
                n179 = call <userlib>:"Write Panel to INI__ogtk.vi"("error in (no error)"=w293, "VI ref"=w287, "refnum"=w294) -> ("error out"=w291:errorcluster, "refnum out"=w292:T2)  [unwired: 7 in]
                n180 = call <vilib>:"Close Config Data.vi"("error in (no error)"=w291, "refnum"=w292) -> ("error out"=w283:errorcluster, "file path"=w284:path)  [unwired: 8 in]
                n181 = Open/Create/Replace File(file path (use dialog)=w284, error in=w283) -> (refnum out=w285:refnum<file>, error out=w286:errorcluster)  [unwired: 4 in, 1 out]
                n182 = Flush File(refnum=w285, error in=w286) -> (refnum out=w281:refnum<file>, error out=w282:errorcluster)
                n183 = Close File(refnum=w281, error in=w282) -> ()  [unwired: 2 out]
              }
            }
            n184 = call "Add State to Queue.vi"("State(s) In (\"\")"=w273) -> ("States Out"=w274:string)  [unwired: 14 in]
          }
          event "盐度补偿": Mouse Down {
            n185 = event-data() -> ("CtlRef"=w298:refnum<vi>)  [unwired: 1 in, 7 out]
            n186 = local read "盐度自动获取"() -> (w299:bool)
            n187 = case shown="假" w299 {
              tunnel: w298 -> [w300 _]
              frame False {
                n188 = property class="DigNum (严格)"(reference=w300) -> (reference out=w301:refnum<vi>, "Value"=w302:dbl)  [unwired: 1 in, 1 out]
                n189 = call "数字键盘.vi"("OldNumber"=w302) -> ("NewNumber"=w303:dbl)  [unwired: 1 in]
                n190 = property class="DigNum (严格)"(reference=w301, "Val(Sgnl)"=w303) -> ()  [unwired: 1 in, 2 out]
              }
              frame True {
              }
            }
            n191 = call "Add State to Queue.vi"("State(s) In (\"\")"=w295) -> ("States Out"=w297:string)  [unwired: 14 in]
          }
          event "校准启动": Value Change {
            n192 = event-data() -> ()  [unwired: 1 in, 6 out]
            n193 = global read "多参数全局变量.vi" "校准运行状态"() -> (w305:T4)
            n194 = Bundle By Name(cluster=w305, "DO"=TRUE) -> (w306:T4)
            n195 = call "Add State to Queue.vi"("State(s) In (\"\")"=w310, "State(s) At Back (\"\")"="init: all\nCal: Place standard solution\n Cal: Calibration process\nidle" ("State(s) In (\"\")")) -> ("States Out"=w309:string)  [unwired: 13 in]
            n196 = global write "多参数全局变量.vi" "校准运行状态"(w306) -> ()
          }
          event "校准停止": Value Change {
            n197 = event-data() -> ()  [unwired: 1 in, 6 out]
            n198 = call "Add State to Queue.vi"("State(s) In (\"\")"="init: all\nCal: Over\nidle" ("State(s) In (\"\")")) -> ("States Out"=w312:string)  [unwired: 14 in]
          }
        }
      }
    }
  }
